vi "rad7maintest.vi"() -> ()   [LabVIEW 2012]
uses:
  <vilib>/Platform/TimedLoop/XDataNode/timing_clust.ctl
  <vilib>/Platform/TimedLoop/XDataNode/nitl_modes.ctl
  <vilib>/Platform/TimedLoop/XDataNode/wakeup.ctl
  <vilib>/Instr/_visa.llb/VISA Configure Serial Port (Instr).vi
  <vilib>/Platform/TimedLoop/XDataNode/XDataNode.xnode
  <vilib>/Platform/TimedLoop/XDataNode/XDNodeRunTimeDep.lvlib
panel:
  out "Rad7 data out":string
  in  "Slow control read rate (Hz)":dbl=1.0
  in  "VISA resource name":refnum<visa-resource-name>
  in  "Loop Time (s)":dbl
  in  "stop":bool
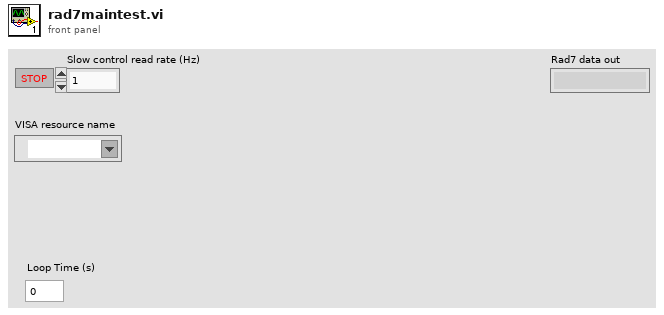
[diagram p1: front panel]
types:
  T1 = typedef "XDNodeRunTimeDep.lvlib/timing_clust.ctl" = cluster{"Expected End [f-1]":u64, "Actual End [f-1]":u64, "Finished Late? [f-1]":bool, "Expected End [i-1]":u64, "Actual End [i-1]":u64, "Finished Late? [i-1]":bool, "Expected Start [i]":u64, "Actual Start [i]":u64, "Expected Start [f]":u64, "Actual Start [f]":u64, "Source Name":string, "Structure Name":string, "Period":i64, "Deadline":i64, "Offset":i64, "Start":i64, "Priority":i32, "Timeout":i32, "Mode":T2, "Wakeup Reason":T3, "Error":errorcluster, "Source Type":string, "Secondary Source Type":string, "Global End Time":u64, "Global Start Time":u64, "Frame Duration":u64, "Iteration Duration":u64, "Assigned CPU":i32, "I/O Scan Engine Mode":u32}
  T2 = typedef "XDNodeRunTimeDep.lvlib/nitl_modes.ctl" = enum32{"No Change", "Process missed periods, maintain original phase", "Discard missed periods, maintain original phase", "Process missed periods, ignore original phase", "Discard missed periods, ignore original phase"}
  T3 = typedef "XDNodeRunTimeDep.lvlib/wakeup.ctl" = enum32{"Normal", "Aborted", "Asynchronous wakeup", "Timing source error", "Timed loop error", "Timeout"}
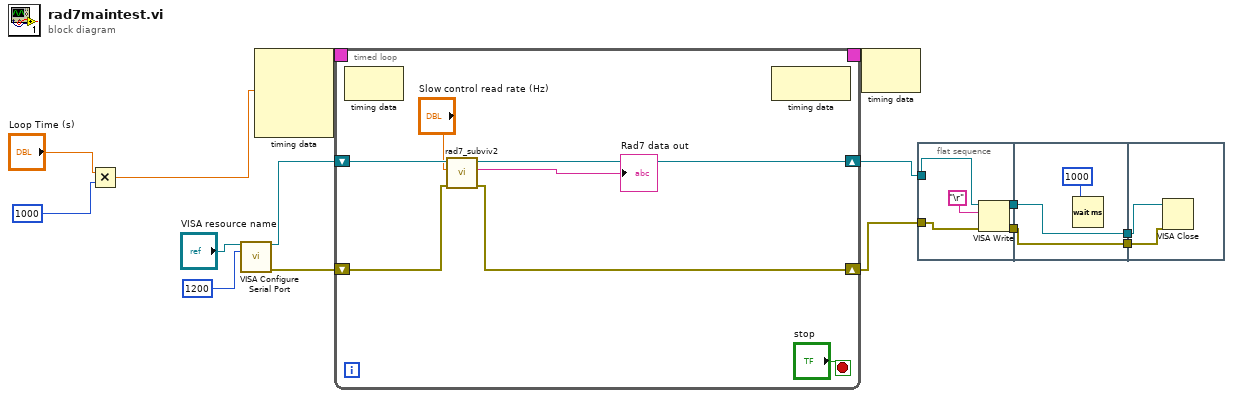
[diagram p0: block diagram]
diagram:
  n1 = Multiply(x="Loop Time (s)", y=1000) -> (x*y=w11:dbl)
  n2 = call-poly "VISA Configure Serial Port"("VISA resource name"="VISA resource name", "baud rate (9600)"=1200) -> ("VISA resource name out"=w8:refnum<visa-resource-name>, "error out"=w7:errorcluster)  [unwired: 12 in]
  n3 = node-c288(w11) -> (w15:T1)  [unwired: 3 in]
  n4 = timed-loop {
    timing: w15 -> [_]
    timing-out: [_] -> w14
    shift-right: [w18] -> w2
    shift-left: w8 -> [w21]
    shift-right: [w17] -> w1
    shift-left: w7 -> [w20]
    stop <- "stop" stop-if-true
    n5 = node-c288() -> ()  [unwired: 1 in, 1 out]
    n6 = call "rad7_subviv2.vi"("error in (no error)"=w20, "Slow control read rate (Hz)"="Slow control read rate (Hz)", "VISA resource name"=w21) -> ("error out"=w17:errorcluster, "Rad7 data out"=→"Rad7 data out":string, "VISA resource name out"=w18:refnum<visa-resource-name>)  [unwired: 4 in, 2 out]
    n7 = node-c288() -> ()  [unwired: 1 in, 1 out]
  }
  n8 = node-c288(w14) -> ()  [unwired: 1 out]
  n9 = flat-sequence {
    tunnel: w1 -> [w28]
    tunnel: w2 -> [w27]
    tunnel: [w26] -> w6
    tunnel: [w25] -> w5
    tunnel: [w31] -> w4
    tunnel: w6 -> [w31]
    tunnel: [w30] -> w3
    tunnel: w5 -> [w30]
    tunnel: w4 -> [w34]
    tunnel: w3 -> [w33]
    frame #0 {
      n10 = VISA Write(VISA resource name=w27, write buffer="\r", error in (no error)=w28) -> (VISA resource name out=w26:refnum<visa-resource-name>, error out=w25:errorcluster)  [unwired: 1 out]
    }
    frame #1 {
      n11 = Wait (ms)(milliseconds to wait=1000) -> ()  [unwired: 1 out]
    }
    frame #2 {
      n12 = VISA Close(VISA resource name=w34, error in (no error)=w33) -> ()  [unwired: 1 out]
    }
  }
